vi "VNA and Keithlay 2400.vi"() -> ()   [LabVIEW 2022 SP3]
uses:
  Keithley 24XX/Public/Data/Read (Single Point).vi
  <vilib>/Utility/file.llb/Write Delimited Spreadsheet (DBL).vi
  Keithley 24XX/Keithley 24XX.lvlib
  Agilent ENA Series/Agilent ENA Series.lvlib
panel:
  in  "Average":i32
  out "Status":sgl
  out "Current":sgl
  out "XY Graph":cluster{dbl[], "Primary / Real":dbl[]}(graph)
  out "Step V":dbl
  in  "Points (>1) V":u32=66
  in  "End V":dbl
  in  "Start V":dbl=-3.0
  in  "VNA VISA resource name":refnum<visa-resource-name>="E5061A"
  in  "Port ( 1)":i32=1
  in  "Measurement Parameters":u16(ring)=1 items=["S11", "S21", "S31", "S41", "S12", "S22", "S32", "S42", "S13", "S23", "S33", "S43", "S14", "S24", "S34", "S44", "A", "B", "C", "D", "R1", "R2", "R3", "R4"]
  in  "Power Level (dBm)":dbl=-5.0 format="%^.2g"
  in  "VNA Points":i32=1000
  in  "Start (Mhz)":dbl=1.0 format="%^.2e"
  in  "Stop (MHz)":dbl=10.0 format="%^.2e"
  in  "Trigger Source":u16(ring) items=["Internal", "External", "Manual", "BUS"]
  in  "Point Trigger (F: Disable)":bool
  in  "Continuous Sweep (T: Enable)":bool=TRUE
  in  "Averaging State (F: Off)":bool
  in  "Average Factor (16)":i32=16
  in  "IF Bandwidth (100000.0)":dbl=1000.0 format="%^.1e"
  in  "Smoothing State (F: Off)":bool
  in  "Wait time (ms)":dbl=4000.0
  in  "file path (dialog if empty)":path=path "C:/Users/B1172_SHG/Documents/NOEMS/test.txt"
  in  "Output Type  (0: Immediate)":u16(ring) items=["Immediate", "Triggered"]
  in  "Source Mode  (0: Voltage)":u16(ring) items=["Voltage", "Current"]
  out "Current Voltage":dbl
  in  "Compliance  Level (0.1)":dbl=0.1
  in  "Keithley VISA resource name":refnum<visa-resource-name>
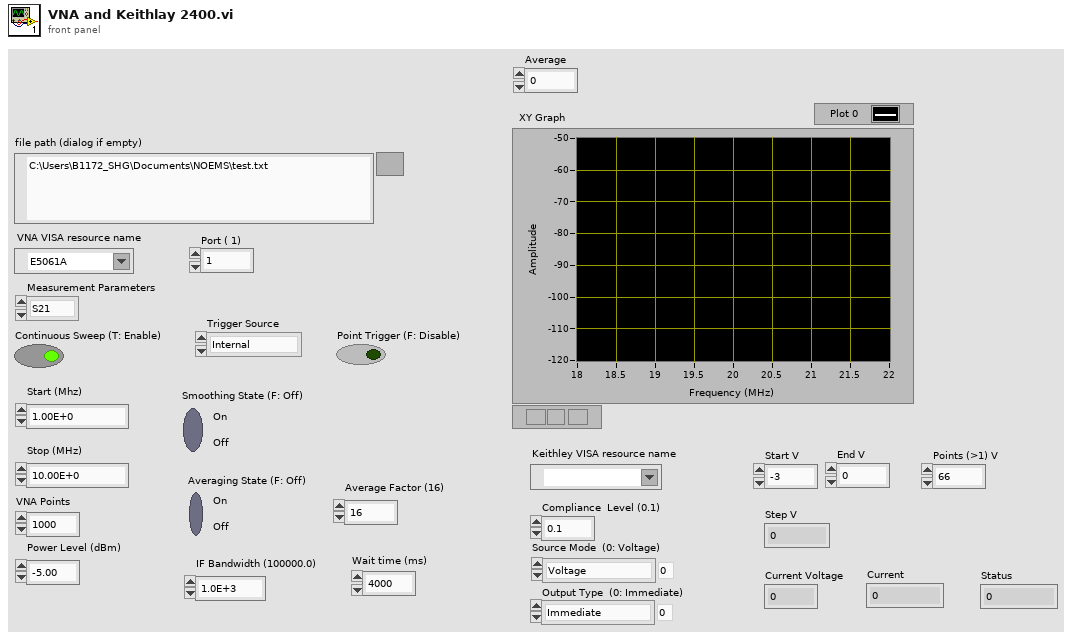
[diagram p1: front panel]
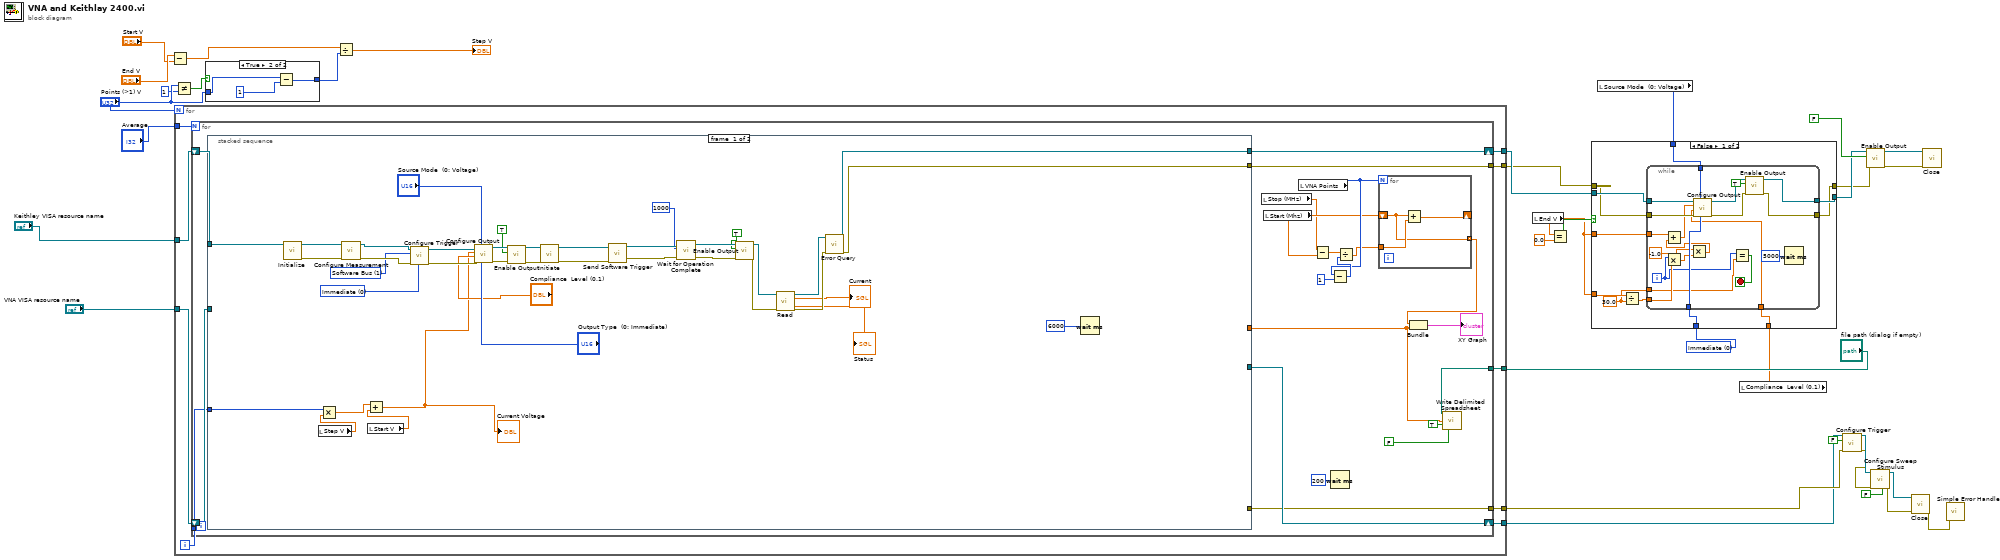
[diagram p0: block diagram]
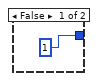
[diagram p3: hidden frame]
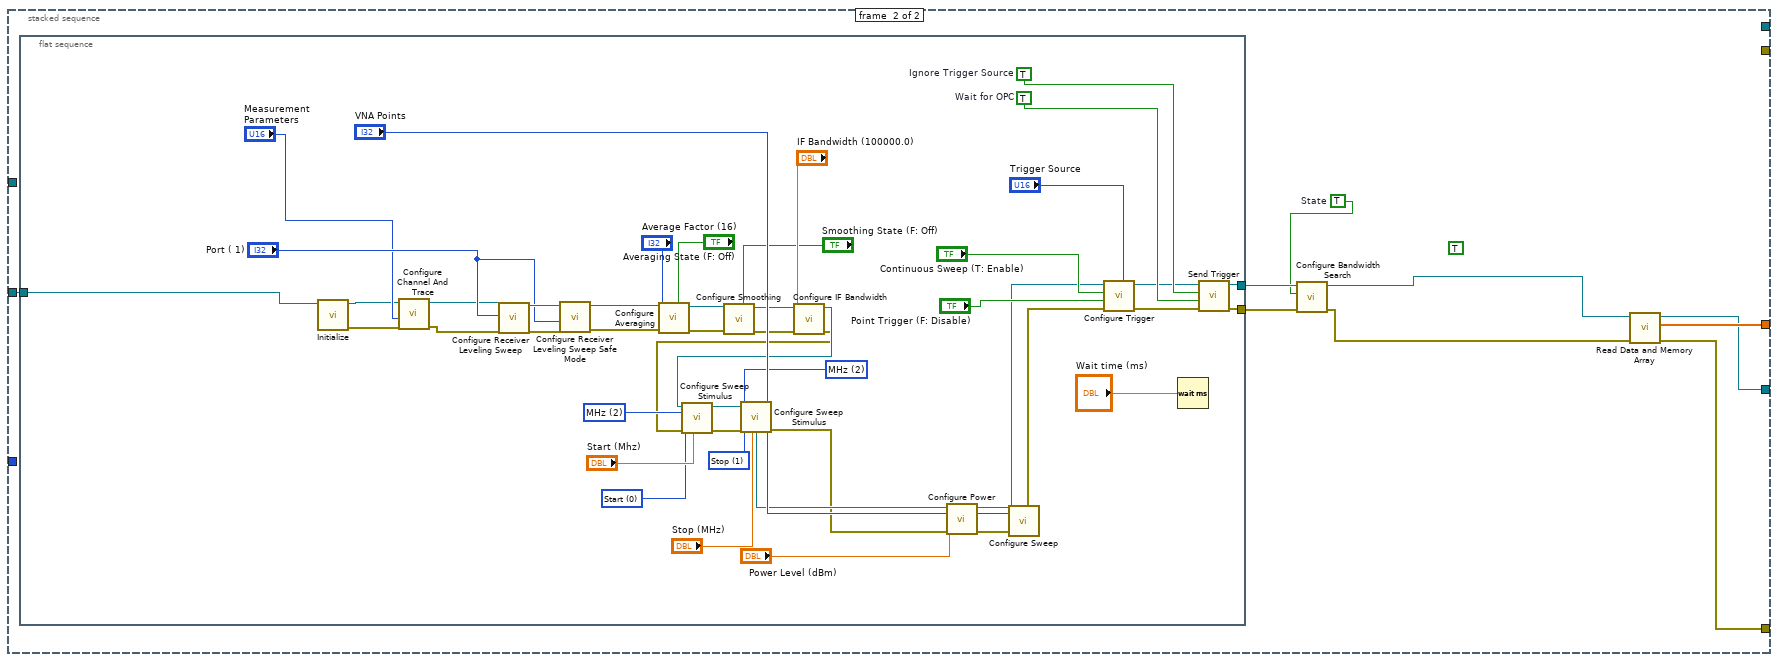
[diagram p4: hidden frame]
diagram:
  w4 = u16 0 items=["Immediate", "Triggered"] ("Output Type  (0: Immediate)")
  n1 = Subtract(x="End V", y="Start V") -> (x-y=w29:dbl)
  n2 = for {
    N: "Points (>1) V" -> [_]
    tunnel: "Keithley VISA resource name" -> [w43]
    tunnel: "VNA VISA resource name" -> [w42]
    tunnel: "file path (dialog if empty)" -> [w41]
    tunnel: [w39] -> w6
    tunnel: [w38] -> w8
    tunnel: [w37] -> w15
    tunnel: [w36] -> w16
    tunnel: "Average" -> [w35]
    i -> [w40]
    n3 = for {
      N: w35 -> [_]
      tunnel: w41 -> [w62]
      tunnel: w40 -> [w58]
      tunnel: [w57] -> w39
      tunnel: [w54] -> w36
      shift-right: [w56] -> w38
      shift-left: w43 -> [w64]
      shift-right: [w55] -> w37
      shift-left: w42 -> [w63]
      n4 = stacked-sequence {
        tunnel: w64 -> [w82 _]
        tunnel: w63 -> [_ w112]
        tunnel: w58 -> [w81 _]
        tunnel: [w76 _] -> w57
        tunnel: [w75 _] -> w56
        tunnel: [_ w107] -> w55
        tunnel: [_ w108] -> w54
        tunnel: [_ w110] -> w52
        frame #0 {
          w86 = u16 1 items=["Immediate", "Software Bus", "Timer", "Manual", "Trigger Link", "Rising SOT Pulse", "Falling SOT Pulse", "Rising or Falling SOT Pulse"] ("Arming Source  (0: Immediate)")
          w87 = u16 0 items=["Immediate", "Trigger Link"] ("Trigger Source (0: Immediate)")
          n5 = call "Initialize.vi"("VISA resource name"=w82) -> ("error out"=w89:errorcluster, "VISA resource name out"=w88:refnum<visa-resource-name>)  [unwired: 9 in]
          n6 = local read "Step V"() -> (w80:dbl)
          n7 = Multiply(x=w81, y=w80) -> (x*y=w79:dbl)
          n8 = call "Configure Measurement.vi"("error in (no error)"=w89, "VISA resource name"=w88) -> ("error out"=w106:errorcluster, "VISA resource name out"=w105:refnum<visa-resource-name>)  [unwired: 8 in]
          n9 = local read "Start V"() -> (w78:dbl)
          n10 = Add(x=w79, y=w78) -> (x+y=w77:dbl)
          "Current Voltage" <- w77
          n11 = call "Configure Trigger.vi"("Trigger Source (0: Immediate)"=w87, "error in (no error)"=w106, "Arming Source  (0: Immediate)"=w86, "VISA resource name"=w105) -> ("error out"=w104:errorcluster, "VISA resource name out"=w103:refnum<visa-resource-name>)  [unwired: 6 in]
          n12 = call "Configure Output.vi"("Output Type  (0: Immediate)"="Output Type  (0: Immediate)", "Source Mode  (0: Voltage)"="Source Mode  (0: Voltage)", "error in (no error)"=w104, "Compliance  Level (0.1)"="Compliance  Level (0.1)", "Output Level (0)"=w77, "VISA resource name"=w103) -> ("error out"=w91:errorcluster, "VISA resource name out"=w90:refnum<visa-resource-name>)  [unwired: 4 in]
          n13 = call "Enable Output.vi"("error in (no error)"=w91, "Enable Output (T: Enable)"=TRUE, "VISA resource name"=w90) -> ("error out"=w93:errorcluster, "VISA resource name out"=w92:refnum<visa-resource-name>)  [unwired: 7 in]
          n14 = call "Initiate.vi"("error in (no error)"=w93, "VISA resource name"=w92) -> ("error out"=w95:errorcluster, "VISA resource name out"=w94:refnum<visa-resource-name>)  [unwired: 8 in]
          n15 = call "Send Software Trigger.vi"("error in (no error)"=w95, "VISA resource name"=w94) -> ("error out"=w100:errorcluster, "VISA resource name out"=w99:refnum<visa-resource-name>)  [unwired: 8 in]
          n16 = call "Wait for Operation Complete.vi"("error in (no error)"=w100, "Timeout (10000 ms)"=u32 1000, "VISA resource name"=w99) -> ("error out"=w102:errorcluster, "VISA resource name out"=w101:refnum<visa-resource-name>)  [unwired: 7 in]
          n17 = call "Enable Output.vi"("error in (no error)"=w102, "Enable Output (T: Enable)"=TRUE, "VISA resource name"=w101) -> ("error out"=w71:errorcluster, "VISA resource name out"=w73:refnum<visa-resource-name>)  [unwired: 7 in]
          n18 = call-poly "Read.vi"("VISA resource name"=w73, "error in (no error)"=w71) -> ("VISA resource name out"=w72:refnum<visa-resource-name>, "Current"=→"Current":sgl, "Status"=→"Status":sgl, "error out"=w70:errorcluster)  [unwired: 7 in, 3 out]
          n19 = call "Error Query.vi"("error in (no error)"=w70, "VISA resource name"=w72) -> ("error out"=w76:errorcluster, "VISA resource name out"=w75:refnum<visa-resource-name>)  [unwired: 6 in, 2 out]
          n20 = Wait (ms)(milliseconds to wait=u32 6000) -> ()  [unwired: 1 out]
        }
        frame #1 {
          w114 = TRUE  # State
          (unwired) TRUE ("Continuous Sweep (T: Enable)")
          n21 = flat-sequence {
            tunnel: [w160] -> w115
            tunnel: [w118] -> w113
            tunnel: w112 -> [w116]
            frame #0 {
              w145 = u16 2 items=["Hz", "kHz", "MHz", "GHz", "dBm", "s", "V"] ("Unit (0: Hz)")
              w146 = u16 2 items=["Hz", "kHz", "MHz", "GHz", "dBm", "s", "V"] ("Unit (0: Hz)")
              w147 = u16 1 items=["Start", "Stop", "Center", "Span"] ("Stimulus (0: Start)")
              w148 = u16 0 items=["Start", "Stop", "Center", "Span"] ("Stimulus (0: Start)")
              w161 = TRUE  # Wait for OPC
              w162 = TRUE  # Ignore Trigger Source
              n22 = call "Initialize.vi"("VISA resource name"=w116) -> ("error out"=w130:errorcluster, "VISA resource name out"=w134:refnum<visa-resource-name>)  [unwired: 9 in]
              n23 = call "Configure Channel And Trace.vi"("error in (no error)"=w130, "Measurement Parameters (0: S11)"="Measurement Parameters", "VISA resource name"=w134) -> ("error out"=w129:errorcluster, "VISA resource name out"=w133:refnum<visa-resource-name>)  [unwired: 7 in]
              n24 = call "Configure Receiver Leveling Sweep.vi"("VISA resource name"=w133, "Port ( 1)"="Port ( 1)", "error in (no error)"=w129) -> ("VISA resource name out"=w158:refnum<visa-resource-name>, "error out"=w128:errorcluster)  [unwired: 15 in]
              n25 = call "Configure Receiver Leveling Sweep Safe Mode.vi"("error in (no error)"=w128, "Port ( 1)"="Port ( 1)", "VISA resource name"=w158) -> ("error out"=w127:errorcluster, "VISA resource name out"=w132:refnum<visa-resource-name>)  [unwired: 7 in]
              n26 = call "Configure Averaging.vi"("Averaging State (F: Off)"="Averaging State (F: Off)", "error in (no error)"=w127, "Factor (16)"="Average Factor (16)", "VISA resource name"=w132) -> ("error out"=w126:errorcluster, "VISA resource name out"=w141:refnum<visa-resource-name>)  [unwired: 6 in]
              n27 = call "Configure Smoothing.vi"("Smoothing State (F: Off)"="Smoothing State (F: Off)", "error in (no error)"=w126, "VISA resource name"=w141) -> ("error out"=w125:errorcluster, "VISA resource name out"=w140:refnum<visa-resource-name>)  [unwired: 7 in]
              n28 = call "Configure IF Bandwidth.vi"("error in (no error)"=w125, "IF Bandwidth (100000.0)"="IF Bandwidth (100000.0)", "VISA resource name"=w140) -> ("error out"=w124:errorcluster, "VISA resource name out"=w139:refnum<visa-resource-name>)  [unwired: 7 in]
              n29 = call "Configure Sweep Stimulus.vi"("Parameter (0.0)"="Start (Mhz)", "error in (no error)"=w124, "Stimulus (0: Start)"=w148, "Unit (0: Hz)"=w146, "VISA resource name"=w139) -> ("error out"=w123:errorcluster, "VISA resource name out"=w152:refnum<visa-resource-name>)  [unwired: 5 in]
              n30 = call "Configure Sweep Stimulus.vi"("Parameter (0.0)"="Stop (MHz)", "error in (no error)"=w123, "Stimulus (0: Start)"=w147, "Unit (0: Hz)"=w145, "VISA resource name"=w152) -> ("error out"=w122:errorcluster, "VISA resource name out"=w151:refnum<visa-resource-name>)  [unwired: 5 in]
              n31 = call "Configure Power.vi"("VISA resource name"=w151, "Power Level (0.0)"="Power Level (dBm)", "error in (no error)"=w122) -> ("VISA resource name out"=w154:refnum<visa-resource-name>, "error out"=w121:errorcluster)  [unwired: 11 in]
              n32 = call "Configure Sweep.vi"("VISA resource name"=w154, "Number of Measurement Points (201)"="VNA Points", "error in (no error)"=w121) -> ("VISA resource name out"=w131:refnum<visa-resource-name>, "error out"=w120:errorcluster)  [unwired: 11 in]
              n33 = call "Configure Trigger.vi"("Trigger Source (0: Internal)"="Trigger Source", "error in (no error)"=w120, "Point Trigger (F: Disable)"="Point Trigger (F: Disable)", "Continuous Sweep (T: Enable)"="Continuous Sweep (T: Enable)", "VISA resource name"=w131) -> ("error out"=w119:errorcluster, "VISA resource name out"=w159:refnum<visa-resource-name>)  [unwired: 5 in]
              n34 = Wait (ms)(milliseconds to wait="Wait time (ms)") -> ()  [unwired: 1 out]
              n35 = call "Send Trigger.vi"("error in (no error)"=w119, "Wait for OPC (F: Do not Wait)"=w161, "Ignore Trigger Source (F: Do not Ignore)"=w162, "VISA resource name"=w159) -> ("error out"=w118:errorcluster, "VISA resource name out"=w160:refnum<visa-resource-name>)  [unwired: 6 in]
            }
          }
          n36 = call "Configure Bandwidth Search.vi"("error in (no error)"=w113, "Result Display State (F: Disable)"=w114, "VISA resource name"=w115) -> ("error out"=w109:errorcluster, "VISA resource name out"=w111:refnum<visa-resource-name>)  [unwired: 7 in]
          n37 = call "Read Data and Memory Array.vi"("error in (no error)"=w109, "VISA resource name"=w111) -> ("error out"=w108:errorcluster, "Primary / Real"=w110:dbl[], "VISA resource name out"=w107:refnum<visa-resource-name>)  [unwired: 6 in, 1 out]
        }
      }
      n38 = local read "Stop (MHz)"() -> (w46:dbl)
      n39 = local read "Start (Mhz)"() -> (w47:dbl)
      n40 = local read "VNA Points"() -> (w50:i32)
      n41 = Subtract(x=w46, y=w47) -> (x-y=w48:dbl)
      n42 = Subtract(x=w50, y=1) -> (x-y=w51:i32)
      n43 = Wait (ms)(milliseconds to wait=u32 200) -> ()  [unwired: 1 out]
      n44 = Divide(x=w48, y=w51) -> (x/y=w49:dbl)
      n45 = for {
        N: w50 -> [_]
        shift-right: [w67] -> _
        shift-left: w47 -> [w65]
        tunnel: w49 -> [w66]
        tunnel: [w65] -> w44 mode=indexing
        n46 = Add(x=w65, y=w66) -> (x+y=w67:dbl)
      }
      n47 = Bundle(w44, "Primary / Real"=w52) -> (→"XY Graph":cluster{dbl[], "Primary / Real":dbl[]})  [unwired: 1 in]
      n48 = call-poly <vilib>:"Write Delimited Spreadsheet.vi"("file path (dialog if empty)"=w62, "1D data"=w52, "append to file? (new file:F)"=TRUE, "transpose? (no:F)"=FALSE) -> ()  [unwired: 10 in, 2 out]
    }
  }
  n49 = Not Equal?(x="Points (>1) V", y=u32 1) -> (x != y?=w25:bool)
  n50 = case shown="True" w25 {
    tunnel: [1 w165] -> w27
    tunnel: "Points (>1) V" -> [_ w164]
    frame False {
    }
    frame True {
      n51 = Subtract(x=w164, y=u32 1) -> (x-y=w165:u32)
    }
  }
  n52 = Divide(x=w29, y=w27) -> (x/y=→"Step V":dbl)
  n53 = local read "End V"() -> (w1:dbl)
  n54 = Equal?(x=w1, y=0.0) -> (x = y?=w10:bool)
  n55 = local read "Source Mode  (0: Voltage)"() -> (w3:u16)
  n56 = local read "Compliance  Level (0.1)"() -> (w2:dbl)
  n57 = case shown="False" w10 {
    tunnel: w8 -> [w173 w199]
    tunnel: [w174 w199] -> w7
    tunnel: w6 -> [w172 w198]
    tunnel: [w171 w198] -> w5
    tunnel: w1 -> [w177 _]
    tunnel: w4 -> [w176 _]
    tunnel: w3 -> [w175 _]
    tunnel: w2 -> [w170 _]
    tunnel: w1 -> [w169 _]
    frame False {
      w168 = 30.0 ("y")
      n58 = Divide(x=w177, y=w168) -> (x/y=w167:dbl)
      n59 = while {
        tunnel: w176 -> [w197]
        tunnel: w173 -> [w196]
        tunnel: w175 -> [w195]
        tunnel: [w185] -> w174
        tunnel: w172 -> [w194]
        tunnel: [w184] -> w171
        tunnel: w167 -> [w192]
        tunnel: w170 -> [w193]
        tunnel: w169 -> [w191]
        tunnel: w168 -> [w178]
        i -> [w179]
        stop <- w187 stop-if-true
        n60 = Multiply(x=w179, y=w192) -> (x*y=w190:dbl)
        n61 = Multiply(x=-1.0, y=w190) -> (x*y=w189:dbl)
        n62 = Add(x=w191, y=w189) -> (x+y=w180:dbl)
        n63 = call "Configure Output.vi"("Output Type  (0: Immediate)"=w197, "Source Mode  (0: Voltage)"=w195, "error in (no error)"=w194, "Compliance  Level (0.1)"=w193, "Output Level (0)"=w180, "VISA resource name"=w196) -> ("error out"=w183:errorcluster, "VISA resource name out"=w186:refnum<visa-resource-name>)  [unwired: 4 in]
        n64 = Equal?(x=w179, y=w178) -> (x = y?=w187:bool)
        n65 = call "Enable Output.vi"("error in (no error)"=w183, "Enable Output (T: Enable)"=TRUE, "VISA resource name"=w186) -> ("error out"=w184:errorcluster, "VISA resource name out"=w185:refnum<visa-resource-name>)  [unwired: 7 in]
        n66 = Wait (ms)(milliseconds to wait=u32 5000) -> ()  [unwired: 1 out]
      }
    }
    frame True {
    }
  }
  n67 = call "Configure Trigger.vi"("error in (no error)"=w16, "Continuous Sweep (T: Enable)"=FALSE, "VISA resource name"=w15) -> ("error out"=w13:errorcluster, "VISA resource name out"=w14:refnum<visa-resource-name>)  [unwired: 7 in]
  n68 = call "Enable Output.vi"("error in (no error)"=w5, "Enable Output (T: Enable)"=FALSE, "VISA resource name"=w7) -> ("error out"=w21:errorcluster, "VISA resource name out"=w22:refnum<visa-resource-name>)  [unwired: 7 in]
  n69 = call "Configure Sweep Stimulus.vi"("Signal Output (T: On)"=FALSE, "error in (no error)"=w13, "VISA resource name"=w14) -> ("error out"=w18:errorcluster, "VISA resource name out"=w19:refnum<visa-resource-name>)  [unwired: 7 in]
  n70 = call "Close.vi"("error in (no error)"=w18, "VISA resource name"=w19) -> ("error out"=w23:errorcluster)  [unwired: 9 in]
  n71 = call "Close.vi"("error in (no error)"=w21, "VISA resource name"=w22) -> ()  [unwired: 9 in, 1 out]
  n72 = call <vilib>:"Simple Error Handler.vi"("error in (no error)"=w23) -> ()  [unwired: 4 in, 5 out]
